vi "Fill Test Names.vi"(8 "error in (no error)":errorcluster, 11 "Test Selector in":refnum<class "Test Selector.lvclass">) -> (0 "error out":errorcluster, 3 "Test Selector out":refnum<class "Test Selector.lvclass">)   [LabVIEW 2019, in "Test Selector.lvlib" / "Test Selector.lvclass"]
uses:
  Test Selector.lvclass
  Test Selector.lvclass/Test Selector.ctl
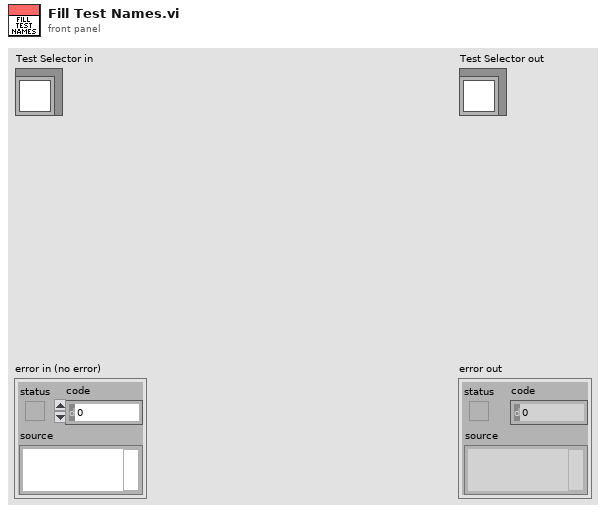
[diagram p1: front panel]
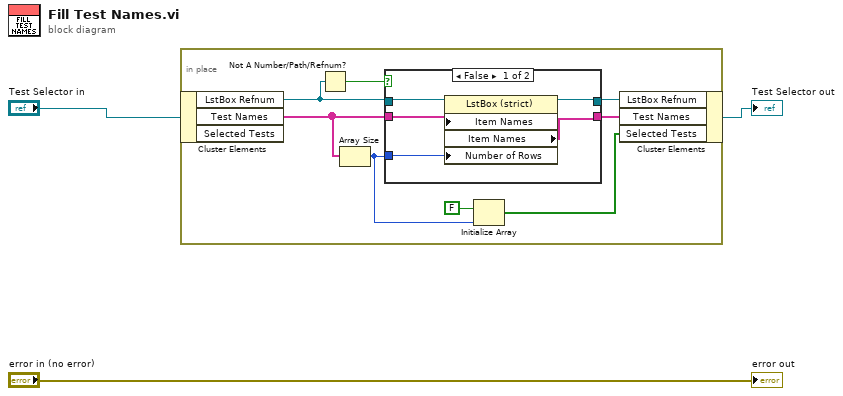
[diagram p0: block diagram]
diagram:
  n1 = in-place {
    n2 = in-place-cluster #1("Test Selector in") -> ("LstBox Refnum"=w10:refnum<vi>, "Test Names"=w7:string[])  [unwired: 1 out]
    n3 = Not A Number/Path/Refnum?(number/path/refnum=w10) -> (NaN/Path/Refnum?=w9:bool)
    n4 = Array Size(array=w7) -> (size(s)=w6:i32)
    n5 = case shown="False" w9 {
      tunnel: [w16 w18] -> w11
      tunnel: w10 -> [w15 w18]
      tunnel: w7 -> [w13 w17]
      tunnel: [w14 w17] -> w8
      tunnel: w6 -> [w12 _]
      frame False {
        n6 = property class="LstBox (strict)"(reference=w15, "Item Names"=w13, "Number of Rows"=w12) -> (reference out=w16:refnum<vi>, "Item Names"=w14:string[])  [unwired: 1 in, 1 out]
      }
      frame True {
      }
    }
    n7 = Initialize Array(FALSE, w6) -> (w4:bool[])
    n8 = in-place-cluster #1("LstBox Refnum"=w11, "Test Names"=w8, "Selected Tests"=w4) -> (→"Test Selector out":refnum<class "Test Selector.lvclass">)
  }
  "error out" <- "error in (no error)"
